vi "Timer_Close.vi"(11 "TIMER":T1 {"Accumulated TIme" format="%13.5p"; "StartTime" format="%13.5p"}) -> ()   [LabVIEW 2019, in "Trajectory_Library.lvlib"]
doc: "Releases resources used by a Timer data cluster. Specifically the semaphore is deleted.\n\nInputs:\n - Timer -- The Timer data cluster"
uses:
  Trajectory_Library.lvlib
  TypeDef/TIMER.ctl
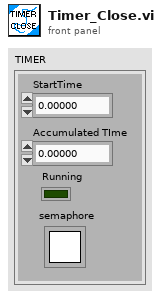
[diagram p1: front panel]
types:
  T1 = typedef "Trajectory_Library.lvlib/TIMER.ctl" = cluster{"StartTime":dbl, "Accumulated TIme":dbl, "Running":bool, "semaphore":T2}
  T2 = typedef "Semaphore RefNum" = refnum<k1>
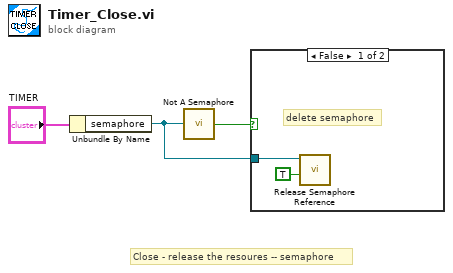
[diagram p0: block diagram]
diagram:
  # "Close - release the resoures -- semaphore"
  n1 = Unbundle By Name("TIMER") -> ("semaphore"=w1:T2)
  n2 = call <vilib>:"Not A Semaphore.vi"("semaphore"=w1) -> ("not a semaphore"=w2:bool)
  n3 = case shown="False" w2 {
    tunnel: w1 -> [w4 _]
    frame False {
      # "delete semaphore"
      n4 = call <vilib>:"Release Semaphore Reference.vi"("force destroy? (F)"=TRUE, "semaphore"=w4) -> ()  [unwired: 8 in, 2 out]
    }
    frame True {
      # "not a semaphore -- ignore"
    }
  }
